vi "Classes Construction.vi"(6 "class":T2, 7 "error in":errorcluster, 8 "param2":variant, 9 "param1":variant, 10 "objects":T1) -> (0 "error out":errorcluster, 2 "init?":bool, 3 "objects":T1)   [LabVIEW 2011]
uses:
  Controls/Class Labels.ctl
  Controls/Class Objects.ctl
  Modules/File/Configuration/Configuration.lvclass
  Modules/Hardware/Power Supply/Power Supply.lvclass
  Modules/Hardware/NMR/NMR.lvclass
  Modules/File/TDMS/TDMS.lvclass
  Controls/TDMS File Handling.ctl
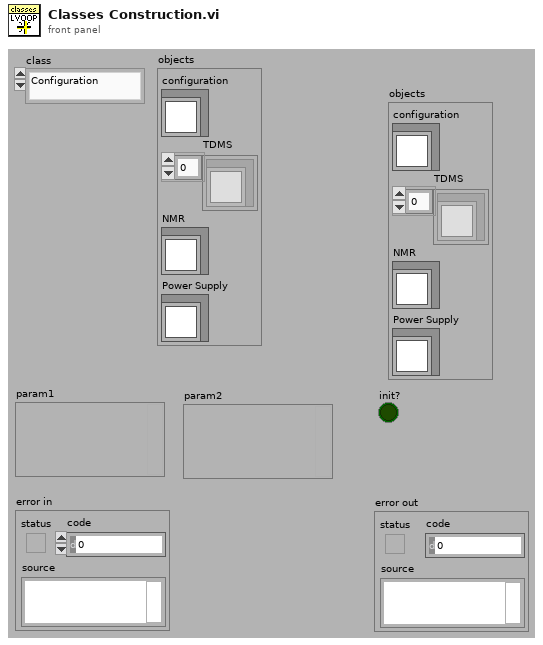
[diagram p1: front panel]
types:
  T1 = typedef "Class Objects.ctl" = cluster{"configuration":refnum<class "Configuration.lvclass">, "TDMS":refnum<class "TDMS.lvclass">[], "Power Supply":refnum<class "Power Supply.lvclass">, "NMR":refnum<class "NMR.lvclass">}
  T2 = typedef "Class Labels.ctl" = enum16{"Configuration", "TDMS", "Detector", "Power Supply", "MFC", "NMR", "Valve Controller"}
  T3 = typedef "TDMS File Handling.ctl" = enum16{"Add TDMS File", "Get Active TDMS File", "Set Active TDMS File", "Set Active TDMS File Index"}
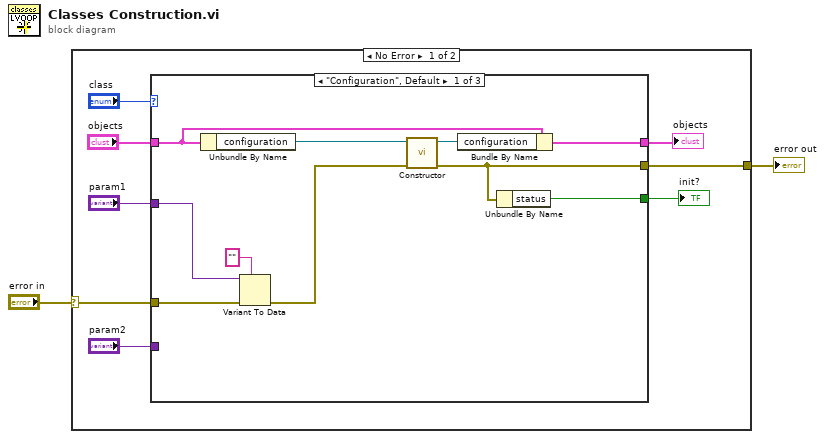
[diagram p0: block diagram]
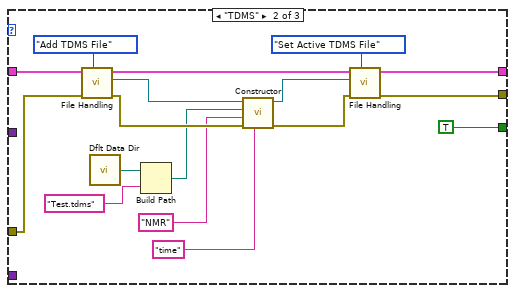
[diagram p2: hidden frame]
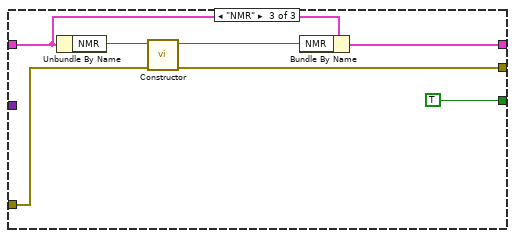
[diagram p3: hidden frame]
diagram:
  n1 = case shown="No Error" "error in" {
    selector: "error in" -> [w7 w45]
    tunnel: [w6 w45] -> w1
    frame No Error {
      n2 = case shown="\"Configuration\", Default" "class" {
        tunnel: "objects" -> [w19 w36 w44]
        tunnel: "param1" -> [w20 _ _]
        tunnel: "param2" -> [_ _ _]
        tunnel: w7 -> [w18 w35 w39]
        tunnel: [w13 w22 w38] -> w6
        tunnel: [w17 w30 w43] -> w3
        tunnel: [w12 TRUE ("status") TRUE ("status")] -> w5
        frame "Configuration", Default {
          n3 = Unbundle By Name(w19) -> ("configuration"=w15:refnum<class "Configuration.lvclass">)
          n4 = Variant To Data(error in=w18, type="", Variant=w20) -> (error out=w14:errorcluster)  [unwired: 1 out]
          n5 = call-dynamic "Constructor.vi"("error in (no error)"=w14, "Configuration in"=w15) -> ("error out"=w13:errorcluster, "Configuration out"=w16:refnum<class "Configuration.lvclass">)  [unwired: 8 in]
          n6 = Bundle By Name(cluster=w19, "configuration"=w16) -> (w17:T1)
          n7 = Unbundle By Name(w13) -> ("status"=w12:bool)
        }
        frame "TDMS" {
          n8 = call "File Handling.vi"("TDMS File Handling"=TDMS_File_Handling."Add TDMS File", "error in"=w35, "objects IN"=w36) -> ("error out"=w29:errorcluster, "TDMS File"=w34:refnum<class "TDMS.lvclass">, "objects OUT"=w31:T1)  [unwired: 6 in]
          n9 = call <vilib>:"Dflt Data Dir.vi"() -> ("App:Default Data Directory"=w27:path)
          n10 = Build Path(base path=w27, name or relative path="Test.tdms") -> (appended path=w25:path)
          n11 = call-dynamic "Constructor.vi"("channel name"="time", "error in"=w29, "group name"="NMR", "path"=w25, "TDMS in"=w34) -> ("error out"=w28:errorcluster, "TDMS out"=w32:refnum<class "TDMS.lvclass">)  [unwired: 5 in]
          n12 = call "File Handling.vi"("TDMS File Handling"=TDMS_File_Handling."Set Active TDMS File", "error in"=w28, "TDMS File"=w32, "objects IN"=w31) -> ("error out"=w22:errorcluster, "objects OUT"=w30:T1)  [unwired: 5 in, 1 out]
        }
        frame "NMR" {
          n13 = Unbundle By Name(w44) -> ("NMR"=w41:refnum<class "NMR.lvclass">)
          n14 = call-dynamic "Constructor.vi"("error in (no error)"=w39, "NMR in"=w41) -> ("error out"=w38:errorcluster, "NMR out"=w40:refnum<class "NMR.lvclass">)  [unwired: 8 in]
          n15 = Bundle By Name(cluster=w44, "NMR"=w40) -> (w43:T1)
        }
      }
      "init?" <- w5
      "objects" <- w3
    }
    frame Error {
    }
  }
  "error out" <- w1
